vi "API - Show Front Panel.vi"(8 "Error In":errorcluster) -> (0 "Error Out":errorcluster)   [LabVIEW 2016, in "Error Manager.lvlib"]
doc: "Displays the Front Panel of the ErrorHandler Main VI to the user.\n\nThe ErrorHandler Main VI (the asynchronous module) must be running when this VI is called.\n\nError in behaviour: This VI executes even if 'error in' contains an error."
uses:
  Error Manager.lvlib
  Queues/MHL Queue/MHL Queue.lvclass
  Queues/MHL Queue/Command (enum).ctl
panel:
  # "Input\nInputs to the VI"
  # "Development\nControls or indicators that are useful for development or testing, but which are not outputs of the VI."
  # "Output\nOutputs of the VI"
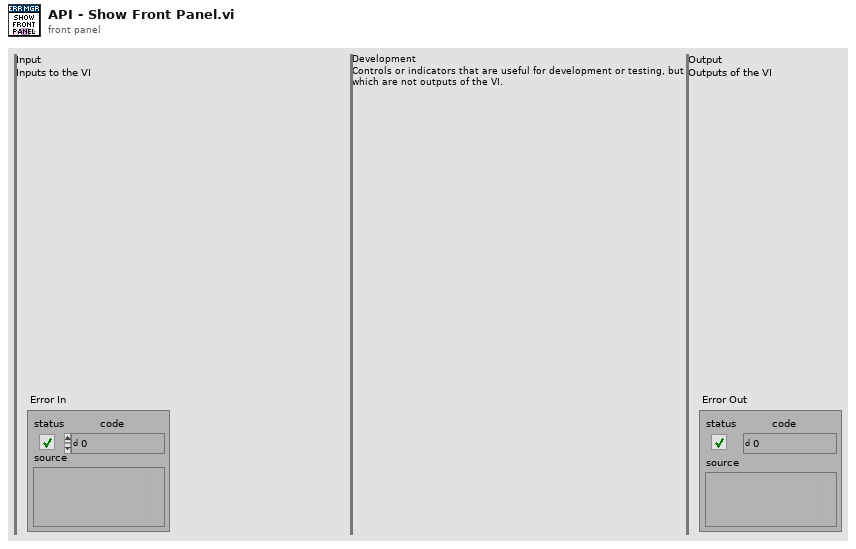
[diagram p1: front panel]
types:
  T1 = typedef "Error Manager.lvlib/MHL Queue.lvclass/Command (enum).ctl" = enum16{"Init Module", "Close Module", "Internal Error", "Create Error Log File", "Show Front Panel", "Handle Error", "Refresh MCL", "MCL Value Change", "Change Display Order", "One-Second Interval Expired", "Mark Selected Errors As Read", "Mark All Errors As Read", "Refresh Button State - MSEAR", "Refresh Button State - MAEAR"}
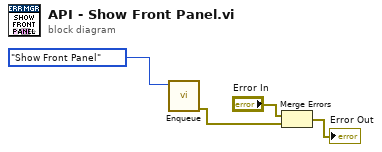
[diagram p0: block diagram]
diagram:
  n1 = call "Enqueue.vi"(11:Command_(enum)."Show Front Panel" ("Command")) -> (0:w3:errorcluster)  [unwired: 10 in]
  n2 = Merge Errors("Error In", w3) -> (→"Error Out":errorcluster)
